vi "Ejercicio_2_1.vi"() -> ()   [LabVIEW 2020]
panel:
  in  "Cantidad de números":i32
  out "Serie":i32[](array[numeric])
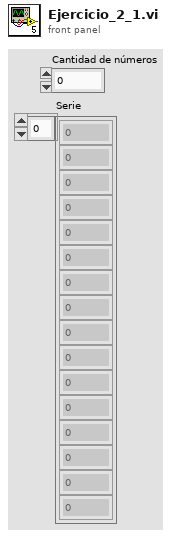
[diagram p1: front panel]
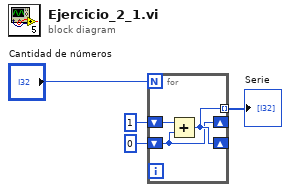
[diagram p0: block diagram]
diagram:
  n1 = for {
    N: "Cantidad de números" -> [_]
    shift-right: [w5] -> _
    shift-left: 1 -> [w7]
    shift-right: [w6] -> _
    shift-left: 0 -> [w5]
    tunnel: [w6] -> w2 mode=indexing
    n2 = Add(x=w7, y=w5) -> (x+y=w6:i32)
  }
  "Serie" <- w2
